vi "Resource to String.vi"(8 "error in (no error)":errorcluster, 10 "Resource as Variant":variant, 11 "LC Parser in":refnum<class "LC Parser.lvclass">) -> (0 "error out":errorcluster, 2 "Resource as String":string, 3 "LC Parser out":refnum<class "LC Parser.lvclass">)   [LabVIEW 2020, in "LC Parser.lvclass"]
uses:
  LC Parser.lvclass
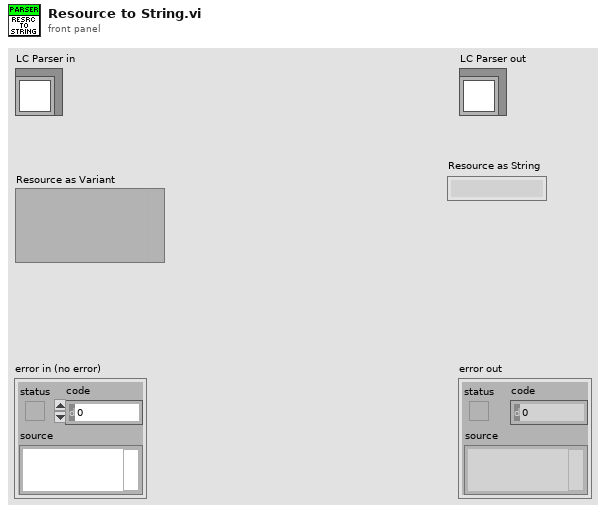
[diagram p1: front panel]
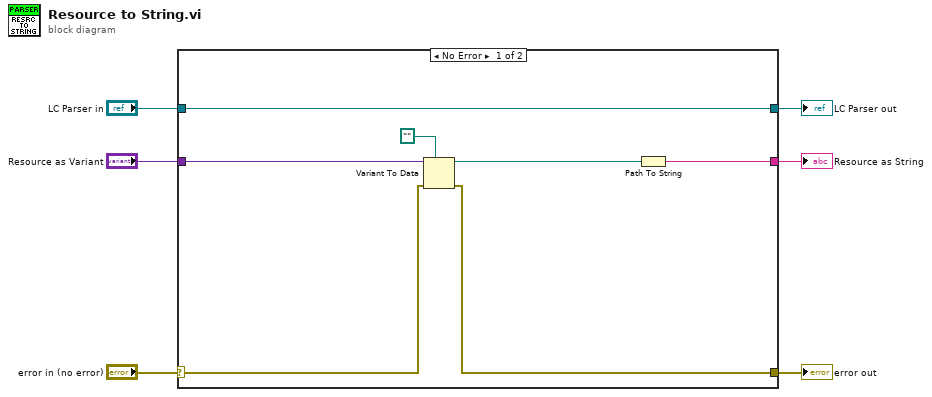
[diagram p0: block diagram]
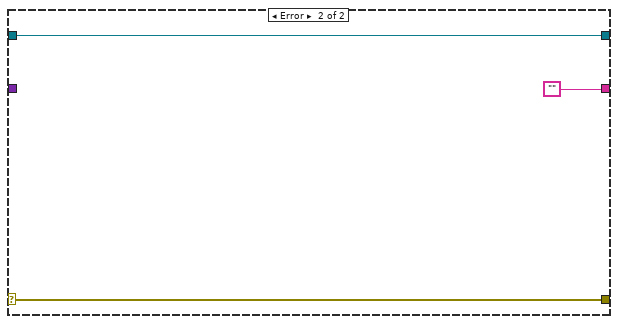
[diagram p2: hidden frame]
diagram:
  n1 = case shown="No Error" "error in (no error)" {
    selector: "error in (no error)" -> [w12 w16]
    tunnel: [w11 w16] -> w6
    tunnel: [w13 w15] -> w4
    tunnel: "LC Parser in" -> [w13 w15]
    tunnel: "Resource as Variant" -> [w10 _]
    tunnel: [w7 ""] -> w5
    frame No Error {
      n2 = Variant To Data(error in=w12, type=path "", Variant=w10) -> (data=w9:path, error out=w11:errorcluster)
      n3 = Path To String(path=w9) -> (string=w7:string)
    }
    frame Error {
    }
  }
  "error out" <- w6
  "LC Parser out" <- w4
  "Resource as String" <- w5
